vi "stringToImage.vi"(6 "label text (image name)":string, 8 "error in (no error)":errorcluster, 9 "Numeric in":dbl, 10 "data out":string, 11 "Refnum in":T1) -> (0 "error out":errorcluster, 1 "Numeric out":dbl, 2 "after substring":string, 3 "Refnum out":T1)   [LabVIEW 2011]
uses:
  IMAQ Image.ctl
panel:
  out "error out 2":errorcluster
  out "bin":i32
  out "NaN/Path/Refnum?":bool
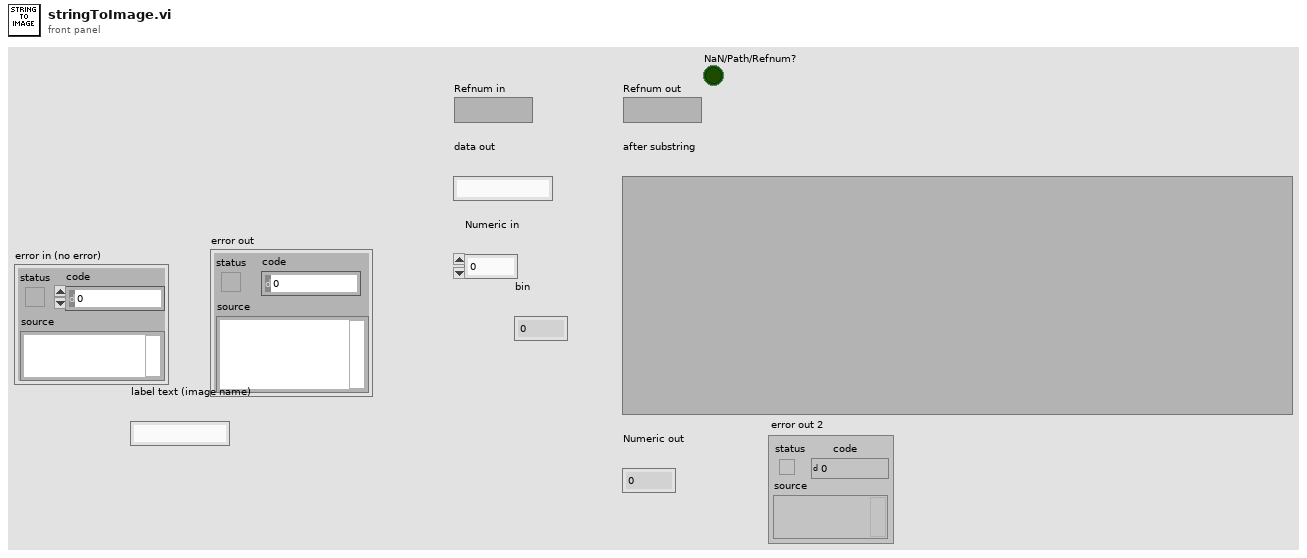
[diagram p1: front panel]
types:
  T1 = typedef "IMAQ Image.ctl" = refnum<image>
  T2 = typedef "Image Type" = u32
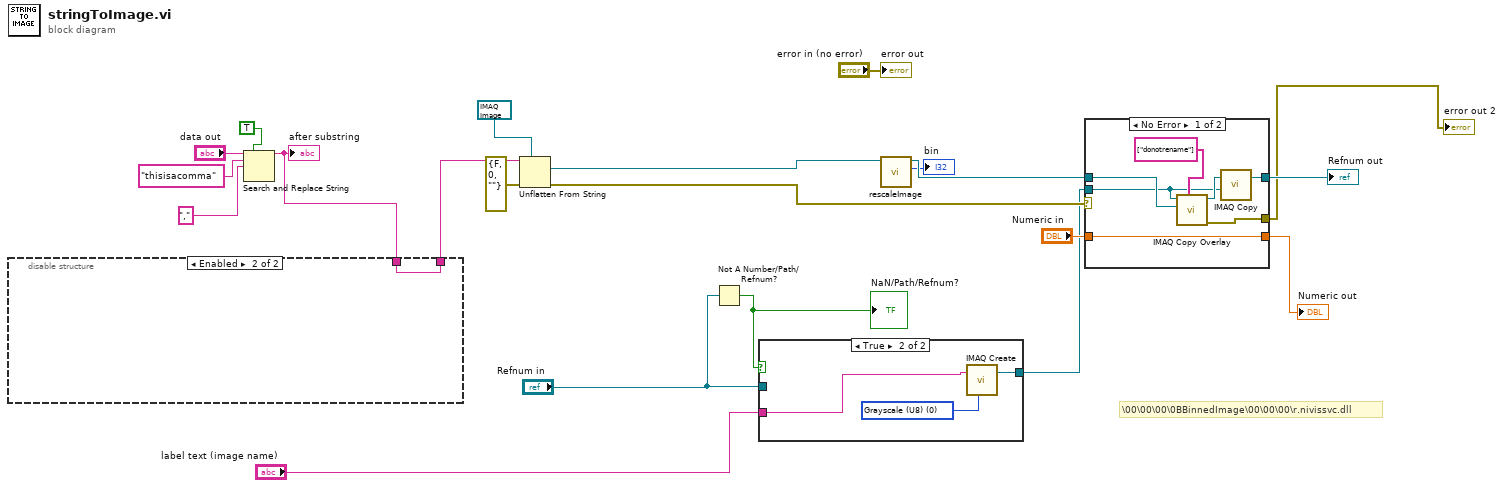
[diagram p0: block diagram]
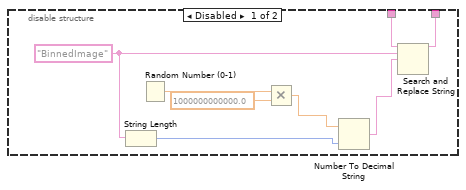
[diagram p2: hidden frame]
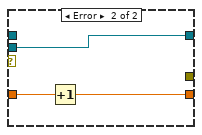
[diagram p4: hidden frame]
diagram:
  # "\\00\\00\\00\\0BBinnedImage\\00\\00\\00\\r.nivissvc.dll"
  n1 = Search and Replace String(replace all?=TRUE ("replace all? (F)"), input string="data out", search string="thisisacomma", replace string="," ("replace string (\"\")")) -> (result string=w3:string)  [unwired: 4 in, 3 out]
  "after substring" <- w3
  n2 = disable-structure shown="Enabled" {
    disable-tunnel: w3 -> [w29 w30]
    disable-tunnel: [w28 w30] -> w2
    frame Disabled {
      w23 = "BinnedImage" ("search string")
      n3 = String Length(string=w23) -> (length=w22:i32)
      n4 = Random Number (0-1)() -> (number: 0 to 1=w27:dbl)
      n5 = Multiply(x=w27, y=1000000000000.0) -> (x*y=w25:dbl)
      n6 = Number To Decimal String(number=w25, width (-)=w22) -> (decimal integer string=w24:string)
      n7 = Search and Replace String(input string=w29, search string=w23, replace string=w24) -> (result string=w28:string)  [unwired: 5 in, 3 out]
    }
    frame Enabled {
    }
  }
  n8 = Unflatten From String(type=T1 refnum ("New Image 2"), binary string=w2, error in (no error)=errorcluster {"status"=FALSE, "code"=0, "source"=""}) -> (value=w10:T1, error out=w16:errorcluster)  [unwired: 3 out]
  n9 = Not A Number/Path/Refnum?(number/path/refnum="Refnum in") -> (NaN/Path/Refnum?=w12:bool)
  "NaN/Path/Refnum?" <- w12
  n10 = case shown="True" w12 {
    tunnel: "Refnum in" -> [w31 _]
    tunnel: [w31 w34] -> w8
    tunnel: "label text (image name)" -> [_ w32]
    frame False {
    }
    frame True {
      w33 = T2 0 items=["Grayscale (U8)", "Grayscale (I16)", "Grayscale (SGL)", "Complex (CSG)", "RGB (U32)", "HSL (U32)", "RGB (U64)", "Grayscale (U16)"] ("Image Type")
      n11 = call "IMAQ Create"("Image Name"=w32, "Image Type"=w33) -> ("New Image"=w34:T1)  [unwired: 3 in, 1 out]
    }
  }
  n12 = call "rescaleImage.vi"("Refnum in"=w10) -> ("bin"=→"bin":i32, "Refnum out"=w11:T1)  [unwired: 9 in]
  n13 = case shown="No Error" w16 {
    tunnel: w11 -> [w38 _]
    tunnel: [w41 w43] -> w14
    tunnel: "Numeric in" -> [w41 w44]
    tunnel: [w39 w42] -> w7
    tunnel: w8 -> [w35 w42]
    tunnel: [w40 _] -> w4
    frame No Error {
      n14 = call "IMAQ Copy Overlay"("Groups"=string[] ["donotrename"], "Image Dst"=w38, "Image Src"=w35) -> ("error out"=w40:errorcluster, "Image Dst Out"=w37:T1)  [unwired: 7 in]
      n15 = call "IMAQ Copy"("Image Dst"=w35, "Image Src"=w37) -> ("Image Dst Out"=w39:T1)  [unwired: 4 in, 1 out]
    }
    frame Error {
      n16 = Increment(x=w44) -> (x+1=w43:dbl)
    }
  }
  "Refnum out" <- w7
  "Numeric out" <- w14
  "error out 2" <- w4
  "error out" <- "error in (no error)"
